vi "LEBITVacuum.destructor.vi"(0 "i ref in":refnum<vi>, 5 "error in(no error)":errorcluster) -> (19 "error out":errorcluster)   [LabVIEW 2014, in "LEBITVacuum.lvlib"]
doc: "This is the destructor of a class.\n\nLicense Agreement for this software:\n\nCopyright (C)\nGesellschaft für Schwerionenforschung, GSI\nPlanckstr. 1\n64291 Darmstadt\nGermany\n\nContact: D.Beck@gsi.de \n\nThis program is free software; you can redistribute it and/or modify it under the terms of the \nGNU General Public License as published by the Free Software Foundation; either version 2 of \nthe license, or (at your option) any later version.\n\nThis program is distributed in the hope that it will be useful, but WITHOUT ANY WARRANTY; \nwithout even the implied warranty of MERCHANTABILITY or FITNESS FOR A PARTICULAR PURPOSE. See the GNU General License for more details (http://www.gnu.org).\n\nGesellschaft für Schwerionenforschung, GSI\nPlanckstr. 1, 64291 Darmstadt, Germany\nFor all questions and ideas contact: M.Richter@gsi.de, H.Brand@gsi.de or D.Beck@gsi.de.\nLast update: 16-JUN-2004"
uses:
  LEBITVacuum.lvlib
  CS_Core/BaseProcess/BaseProcess.lvlib
  CSlibraries-extern/DimLVEvent/LVDimInterface/LVDimInterface.lvlib
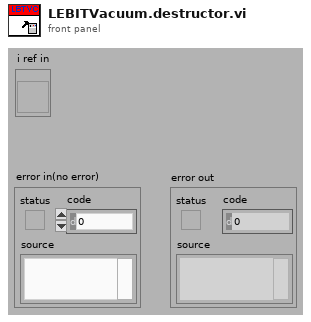
[diagram p1: front panel]
types:
  T1 = typedef "LEBITVacuum.lvlib/LEBITVacuum.i attribute.ctl" = cluster{"setValuePLC":string[], "nickNames":string[], "setValuePLCServiceID":i32[], "monValuePLC":string[], "SetValueServiceID":i32[], "MonValueServiceID":i32[], "SetValue":i16[], "AllPLCValues":string[], "CondSpecial2DArray":string[][], "CondSpecialIndex":i32[], "ReasonForLocking":string, "ReasonForLockingID":i32, "enableValuePLC":string[], "OverwriteCloseSafetyPLC":string[], "OverwriteOpenSafetyPLC":string[], "OverwriteCloseSafetyPLCServiceID":i32[], "OverwriteOpenSafetyPLCServiceID":i32[], "MKS Address Array":i32[][], "MKS MeasurementServiceID":i32[], "MKS Measurement":string[], "CRYO Measurement":string[][], "CRYO MeasurementServiceID":i32[], "Special":string[], "Start Date":string, "MKS VISA resource":refnum<visa-resource-name>, "CRYO VISA resource":refnum<visa-resource-name>}
  T2 = enum16{"SetAttribute", "GetAttribute", "CreateAttribute", "DestroyAttribute", "DestroyAllAtributes"}
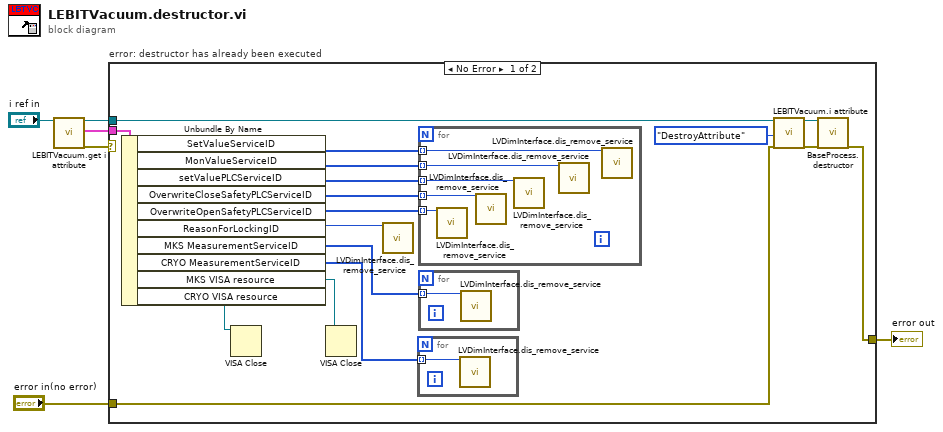
[diagram p0: block diagram]
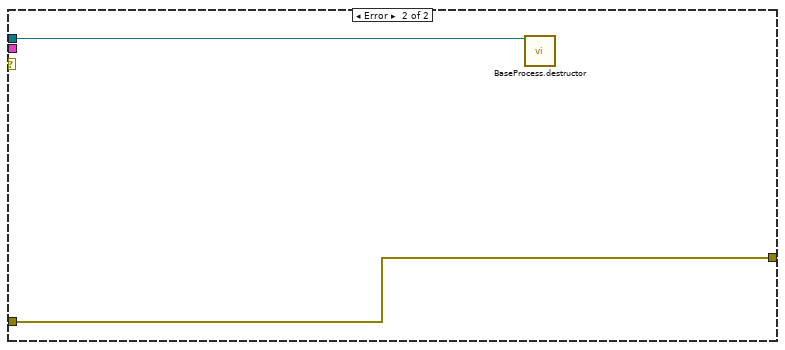
[diagram p2: hidden frame]
diagram:
  n1 = call "LEBITVacuum.get i attribute.vi"("i ref in"="i ref in") -> ("i ref out"=w2:refnum<vi>, "i attribute"=w1:T1, "error out"=w3:errorcluster)  [unwired: 16 in]
  n2 = case "error: destructor has already been executed" shown="No Error" w3 {
    tunnel: [w15 w32] -> w6
    tunnel: "error in(no error)" -> [w14 w32]
    tunnel: w2 -> [w20 w31]
    tunnel: w1 -> [w19 _]
    frame No Error {
      n3 = Unbundle By Name(w19) -> ("SetValueServiceID"=w18:i32[], "MonValueServiceID"=w17:i32[], "setValuePLCServiceID"=w16:i32[], "OverwriteCloseSafetyPLCServiceID"=w13:i32[], "OverwriteOpenSafetyPLCServiceID"=w12:i32[], "ReasonForLockingID"=w11:i32, "MKS MeasurementServiceID"=w10:i32[], "CRYO MeasurementServiceID"=w9:i32[], "MKS VISA resource"=w8:refnum<visa-resource-name>, "CRYO VISA resource"=w7:refnum<visa-resource-name>)
      n4 = VISA Close(VISA resource name=w7) -> ()  [unwired: 1 in, 1 out]
      n5 = VISA Close(VISA resource name=w8) -> ()  [unwired: 1 in, 1 out]
      n6 = call "LVDimInterface.dis_remove_service.vi"("my_serviceID"=w11) -> ()  [unwired: 18 in, 1 out]
      n7 = for {
        tunnel: w9 -> [w24] mode=indexing
        n8 = call "LVDimInterface.dis_remove_service.vi"("my_serviceID"=w24) -> ()  [unwired: 18 in, 1 out]
      }
      n9 = for {
        tunnel: w18 -> [w30] mode=indexing
        tunnel: w17 -> [w29] mode=indexing
        tunnel: w16 -> [w28] mode=indexing
        tunnel: w13 -> [w27] mode=indexing
        tunnel: w12 -> [w26] mode=indexing
        n10 = call "LVDimInterface.dis_remove_service.vi"("my_serviceID"=w26) -> ()  [unwired: 18 in, 1 out]
        n11 = call "LVDimInterface.dis_remove_service.vi"("my_serviceID"=w27) -> ()  [unwired: 18 in, 1 out]
        n12 = call "LVDimInterface.dis_remove_service.vi"("my_serviceID"=w28) -> ()  [unwired: 18 in, 1 out]
        n13 = call "LVDimInterface.dis_remove_service.vi"("my_serviceID"=w29) -> ()  [unwired: 18 in, 1 out]
        n14 = call "LVDimInterface.dis_remove_service.vi"("my_serviceID"=w30) -> ()  [unwired: 18 in, 1 out]
      }
      n15 = for {
        tunnel: w10 -> [w25] mode=indexing
        n16 = call "LVDimInterface.dis_remove_service.vi"("my_serviceID"=w25) -> ()  [unwired: 18 in, 1 out]
      }
      n17 = call "LEBITVacuum.i attribute.vi"("VI Refnum"=w20, "Action"=T2."DestroyAttribute", "error in (no error)"=w14) -> ("VI Refnum out"=w22:refnum<vi>, "error out"=w21:errorcluster)  [unwired: 14 in, 1 out]
      n18 = call "BaseProcess.destructor.vi"("i ref in"=w22, "error in (no error)"=w21) -> ("error out"=w15:errorcluster)  [unwired: 17 in]
    }
    frame Error {
      n19 = call "BaseProcess.destructor.vi"("i ref in"=w31) -> ()  [unwired: 18 in, 1 out]
    }
  }
  "error out" <- w6
